vi "draw.vi"(0 "reference":refnum<class "SegmentedLineEdge.lvclass">, 1 "graphics":refnum<class "Graphics.lvclass">, 5 "error in (no error)":errorcluster) -> (14 "reference out":refnum<class "SegmentedLineEdge.lvclass">, 19 "error out":errorcluster)   [LabVIEW 2014, in "SegmentedLineEdge.lvclass"]
doc: "public void draw(Graphics2D g2)"
uses:
  <resource>/Framework/Providers/Open_GDS/UML/SegmentedLineEdge_class/SegmentedLineEdge.lvclass
  <resource>/Framework/Providers/Open_GDS/UML/Graphics_class/Graphics.lvclass
  <resource>/Framework/Providers/Open_GDS/UML/ClassNode_class/ClassNode.lvclass
  <resource>/Framework/Providers/Open_GDS/UML/Graphics_class/StrokeType.ctl
  <resource>/Framework/Providers/Open_GDS/UML/LineStyle_class/LineStyle.lvclass
  <resource>/Framework/Providers/Open_GDS/UML/ArrowHead_class/ArrowHead.lvclass
  <resource>/Framework/Providers/Open_GDS/UML/MultiLineString_class/MultiLineString.lvclass
  <resource>/Framework/Providers/Open_GDS/UML/AbstractNode_class/AbstractNode.lvclass
  <resource>/Framework/Providers/Open_GDS/UML/AbstractEdge_class/AbstractEdge.lvclass
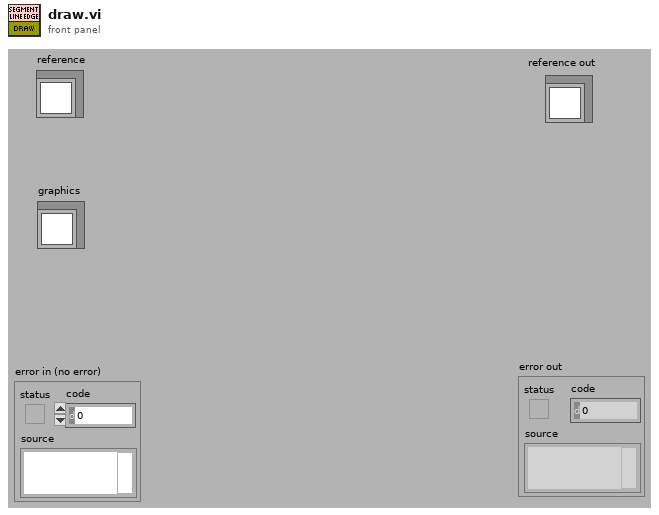
[diagram p1: front panel]
types:
  T1 = typedef "Graphics.lvclass/StrokeType.ctl" = enum16{"USE_DEFAULT", "SOLID", "DOTTED"}
  T2 = typedef "SegmentedLineEdge.lvclass/ObjectAttributes.ctl" = cluster{"lineStyle":refnum<class "LineStyle.lvclass">, "startArrowHead":refnum<class "ArrowHead.lvclass">, "endArrowHead":refnum<class "ArrowHead.lvclass">, "startLabel":string, "midLabel":string, "endLabel":string, "MidLabelOffset":T3, "SplitWire":bool}
  T3 = typedef "Point Point2D.ctl" = cluster{"x":dbl, "y":dbl}
  T4 = typedef "AbstractEdge.lvclass/ObjectAttributes.ctl" = cluster{"start":refnum<class "AbstractNode.lvclass">, "end":refnum<class "AbstractNode.lvclass">}
  T5 = typedef "LineStyle.lvclass/LineStyleType.ctl" = enum16{"SOLID", "DOTTED"}
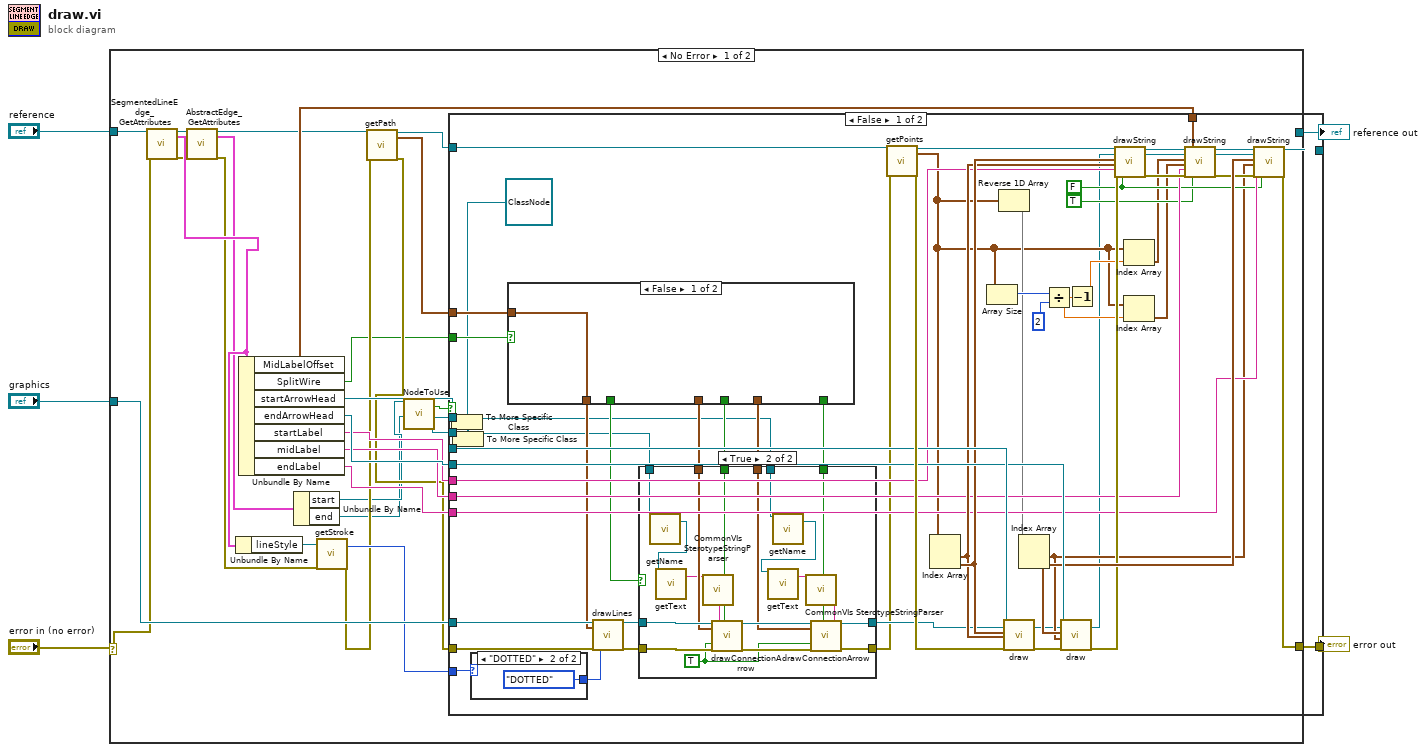
[diagram p0: block diagram]
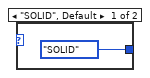
[diagram p2: hidden frame]
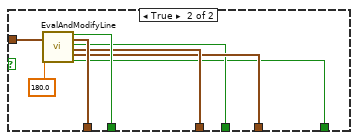
[diagram p3: hidden frame]
diagram:
  n1 = case shown="No Error" "error in (no error)" {
    selector: "error in (no error)" -> [w30 w121]
    tunnel: "reference" -> [w34 w122]
    tunnel: [w33 w121] -> w4
    tunnel: [w32 w122] -> w3
    tunnel: "graphics" -> [w31 _]
    frame No Error {
      n2 = call <resource>:"SegmentedLineEdge_GetAttributes.vi"("reference in"=w34, "error in (no error)"=w30) -> ("reference out"=w10:refnum<class "SegmentedLineEdge.lvclass">, "Data"=w11:T2, "error out"=w9:errorcluster)  [unwired: 1 in, 14 out]
      n3 = call <resource>:"AbstractEdge_GetAttributes.vi"("reference in"=w10, "error in (no error)"=w9) -> ("reference out"=w7:refnum<class "SegmentedLineEdge.lvclass">, "Data"=w6:T4, "error out"=w8:errorcluster)  [unwired: 14 in, 1 out]
      n4 = Unbundle By Name(w11) -> ("lineStyle"=w29:refnum<class "LineStyle.lvclass">)
      n5 = Unbundle By Name(w11) -> ("MidLabelOffset"=w19:T3, "SplitWire"=w17:bool, "startArrowHead"=w27:refnum<class "ArrowHead.lvclass">, "endArrowHead"=w26:refnum<class "ArrowHead.lvclass">, "startLabel"=w25:string, "midLabel"=w24:string, "endLabel"=w23:string)
      n6 = Unbundle By Name(w6) -> ("start"=w16:refnum<class "AbstractNode.lvclass">, "end"=w14:refnum<class "AbstractNode.lvclass">)
      n7 = call-dynamic "getStroke.vi"("reference"=w29, "error in (no error)"=w8) -> ("lineStyle"=w22:T5, "error out"=w21:errorcluster)  [unwired: 15 in, 1 out]
      n8 = call-dynamic "getPath.vi"("reference"=w7, "error in (no error)"=w21) -> ("reference out"=w28:refnum<class "SegmentedLineEdge.lvclass">, "path"=w18:T3[], "error out"=w20:errorcluster)  [unwired: 15 in]
      n9 = call <resource>:"NodeToUse.vi"("reference in"=w16, "reference in 2"=w14) -> ("reference out"=w15:refnum<class "AbstractNode.lvclass">, "Same"=w12:bool, "reference out 2"=w13:refnum<class "AbstractNode.lvclass">)  [unwired: 14 in, 1 out]
      n10 = case shown="False" w12 {
        tunnel: [w86 w119] -> w33
        tunnel: [w85 w120] -> w32
        tunnel: w31 -> [w84 _]
        tunnel: w28 -> [w83 w120]
        tunnel: w27 -> [w81 _]
        tunnel: w26 -> [w79 _]
        tunnel: w25 -> [w73 _]
        tunnel: w24 -> [w68 _]
        tunnel: w23 -> [w67 _]
        tunnel: w22 -> [w36 _]
        tunnel: w20 -> [w55 w119]
        tunnel: w19 -> [w54 _]
        tunnel: w18 -> [w53 _]
        tunnel: w17 -> [w42 _]
        tunnel: w15 -> [w38 _]
        tunnel: w13 -> [w37 _]
        frame False {
          w40 = refnum<class "ClassNode.lvclass"> refnum ("reference")
          w66 = FALSE ("center")
          n11 = To More Specific Class(target class=w40, reference=w38) -> (specific class reference=w41:refnum<class "ClassNode.lvclass">)  [unwired: 1 in, 1 out]
          n12 = To More Specific Class(target class=w40, reference=w37) -> (specific class reference=w39:refnum<class "ClassNode.lvclass">)  [unwired: 1 in, 1 out]
          n13 = case shown="\"DOTTED\"" w36 {
            tunnel: [StrokeType."SOLID" ("stroke") StrokeType."DOTTED" ("stroke")] -> w35
            frame "SOLID", Default {
            }
            frame "DOTTED" {
            }
          }
          n14 = case shown="False" w42 {
            tunnel: w53 -> [w89 w97]
            tunnel: [w89 w96] -> w52
            tunnel: [_ w94] -> w47
            tunnel: [_ w93] -> w46
            tunnel: [_ w92] -> w45
            tunnel: [_ w91] -> w44
            tunnel: [_ w90] -> w43
            frame False {
            }
            frame True {
              n15 = call <resource>:"EvalAndModifyLine.vi"("path 2"=w97, "MaxLength"=180.0) -> ("Ecxeeded"=w94:bool, "path"=w96:T3[], "Point1_Can'tGoLeft"=w91:bool, "Point1"=w93:T3, "PointN-1"=w92:T3, "PointN-1_Can'tGoLeft"=w90:bool)  [unwired: 2 in, 10 out]
            }
          }
          n16 = call <resource>:"drawLines.vi"("reference"=w84, "points"=w52, "error in (no error)"=w55, "stroke"=w35) -> ("reference out"=w51:refnum<class "Graphics.lvclass">, "error out"=w50:errorcluster)  [unwired: 3 in, 11 out]
          n17 = case shown="True" w47 {
            tunnel: w51 -> [w99 w118]
            tunnel: w50 -> [w98 w117]
            tunnel: [w99 w114] -> w49
            tunnel: [w98 w113] -> w48
            tunnel: w46 -> [_ w112]
            tunnel: w45 -> [_ w111]
            tunnel: w39 -> [_ w105]
            tunnel: w41 -> [_ w103]
            tunnel: w43 -> [_ w101]
            tunnel: w44 -> [_ w100]
            frame False {
            }
            frame True {
              w110 = TRUE ("fill?(F)")
              n18 = call-dynamic "getName.vi"("reference"=w105) -> ("name"=w104:refnum<class "MultiLineString.lvclass">)  [unwired: 16 in, 2 out]
              n19 = call-dynamic "getText.vi"("reference"=w104) -> ("text"=w109:string)  [unwired: 16 in, 2 out]
              n20 = call <resource>:"CommonVIs SterotypeStringParser.vi"("SterotypeStringIn"=w109) -> ("Name"=w108:string)  [unwired: 18 out]
              n21 = call <resource>:"drawConnectionArrow.vi"("reference"=w118, "point2D"=w112, "fill?(F)"=w110, "error in (no error)"=w117, "Label"=w108, "Can'tGoLeft"=w100) -> ("reference out"=w115:refnum<class "Graphics.lvclass">, "error out"=w116:errorcluster)  [unwired: 1 in, 11 out]
              n22 = call-dynamic "getName.vi"("reference"=w103) -> ("name"=w102:refnum<class "MultiLineString.lvclass">)  [unwired: 16 in, 2 out]
              n23 = call-dynamic "getText.vi"("reference"=w102) -> ("text"=w107:string)  [unwired: 16 in, 2 out]
              n24 = call <resource>:"CommonVIs SterotypeStringParser.vi"("SterotypeStringIn"=w107) -> ("Name"=w106:string)  [unwired: 18 out]
              n25 = call <resource>:"drawConnectionArrow.vi"("reference"=w115, "point2D"=w111, "fill?(F)"=w110, "error in (no error)"=w116, "Label"=w106, "Can'tGoLeft"=w101) -> ("reference out"=w114:refnum<class "Graphics.lvclass">, "error out"=w113:errorcluster)  [unwired: 1 in, 11 out]
            }
          }
          n26 = call-dynamic "getPoints.vi"("reference"=w83, "error in (no error)"=w48) -> ("reference out"=w76:refnum<class "SegmentedLineEdge.lvclass">, "points"=w59:T3[], "error out"=w82:errorcluster)  [unwired: 15 in]
          n27 = Index Array(array=w59) -> (element #1=w74:T3, element #2=w75:T3)  [unwired: 2 in]
          n28 = Array Size(array=w59) -> (size(s)=w63:i32)
          n29 = Reverse 1D Array(array=w59) -> (reversed array=w60:T3[])
          n30 = call-dynamic "draw.vi"("reference"=w81, "graphics"=w49, "p1"=w75, "p2"=w74, "error in (no error)"=w82) -> ("error out"=w80:errorcluster)  [unwired: 13 in, 1 out]
          n31 = Index Array(array=w60) -> (element #1=w64:T3, element #2=w78:T3)  [unwired: 2 in]
          n32 = Divide(x=w63, y=2) -> (x/y=w58:dbl)
          n33 = call-dynamic "draw.vi"("reference"=w79, "graphics"=w49, "p1"=w78, "p2"=w64, "error in (no error)"=w80) -> ("error out"=w77:errorcluster)  [unwired: 13 in, 1 out]
          n34 = Decrement(x=w58) -> (x-1=w61:dbl)
          n35 = call-dynamic "drawString.vi"("reference"=w76, "graphics"=w49, "p1"=w75, "p2"=w74, "text"=w73, "error in (no error)"=w77, "center"=w66) -> ("reference out"=w72:refnum<class "SegmentedLineEdge.lvclass">, "error out"=w71:errorcluster)  [unwired: 11 in]
          n36 = Index Array(array=w59, index=w61) -> (element=w57:T3)
          n37 = Index Array(array=w59, index=w58) -> (element=w56:T3)
          n38 = call-dynamic "drawString.vi"("reference"=w72, "graphics"=w49, "p1"=w57, "p2"=w56, "text"=w68, "error in (no error)"=w71, "Offset"=w54, "center"=TRUE) -> ("reference out"=w70:refnum<class "SegmentedLineEdge.lvclass">, "error out"=w69:errorcluster)  [unwired: 10 in]
          n39 = call-dynamic "drawString.vi"("reference"=w70, "graphics"=w49, "p1"=w78, "p2"=w64, "text"=w67, "error in (no error)"=w69, "center"=w66) -> ("reference out"=w85:refnum<class "SegmentedLineEdge.lvclass">, "error out"=w86:errorcluster)  [unwired: 11 in]
        }
        frame True {
        }
      }
    }
    frame Error {
    }
  }
  "reference out" <- w3
  "error out" <- w4
